vi "My_Controls_Example.vi"() -> ()   [LabVIEW 2021]
uses:
  <vilib>/addons/Control Design/_Model Construction/Special Model Creation.llb/Special Model Creation SubVI/CD Create 2nd Order Model.vi
  <vilib>/addons/Control Design/_Time Response Analysis/Time Response.llb/Time Response subVI/cd_Step Response (Transfer Function).vi
  <vilib>/addons/Control Design/_Model Construction/NI_CD_Special Model Creation.lvlib
  <vilib>/addons/Control Design/_Time Response Analysis/NI_CD_Time Response.lvlib
panel:
  in  "stop":bool
  out "Step Response Graph":cluster{"time":dbl[], dbl[]}[](graph)
  in  "Natural Frequency":dbl(slide) scale=0.0..5.0
  in  "Damping Ratio":dbl(slide) scale=0.0..1.0
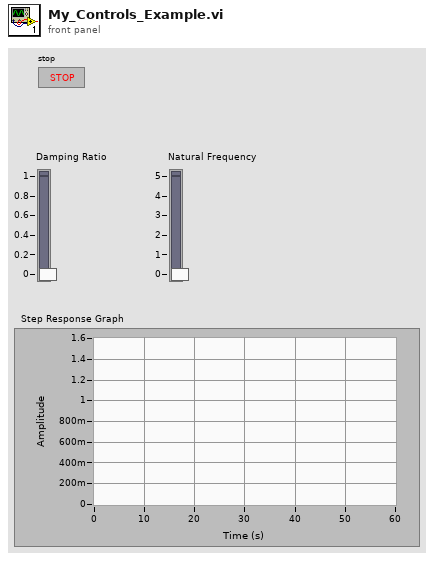
[diagram p1: front panel]
types:
  T1 = typedef "NI_LinSys_Model Typedefs.lvlib/CD Transfer Function Model (MIMO).ctl" = cluster{"properties":T2, "transfer function(s)":T3[][]}
  T2 = typedef "NI_LinSys_Model Typedefs.lvlib/CD General Elements.ctl" = cluster{"Model name":string, "Input names":string[], "Output names":string[], "Input Delays":dbl[], "Output Delays":dbl[], "Sampling Time":dbl, "Notes":string}
  T3 = typedef "NI_LinSys_Model Typedefs.lvlib/CD Transfer Function Model (SISO).ctl" = cluster{"Numerator":dbl[], "Denominator":dbl[], "delay":dbl}
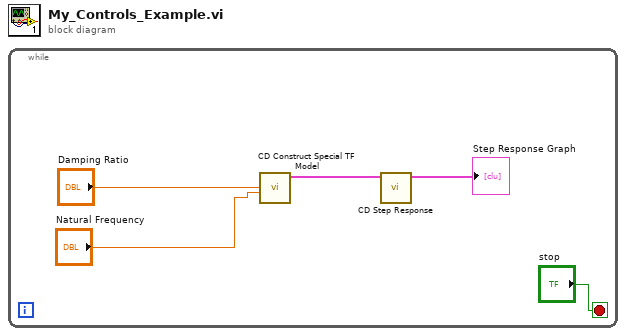
[diagram p0: block diagram]
diagram:
  n1 = while {
    stop <- "stop" stop-if-true
    n2 = call-poly <vilib>:"CD Construct Special TF Model.vi"("Natural Frequency (rad/s)"="Natural Frequency", "Damping Ratio"="Damping Ratio") -> ("Transfer Function Model"=w3:T1)  [unwired: 8 in, 1 out]
    n3 = call-poly <vilib>:"CD Step Response.vi"("Transfer Function Model"=w3) -> ("Step Response Graph"=→"Step Response Graph":cluster{"time":dbl[], dbl[]}[])  [unwired: 8 in, 2 out]
  }
